vi "CLD 2  Elapsed Time Express Caller Exercise.vi"() -> ()   [LabVIEW 2019]
doc: "CLD 2 Exercise"
panel:
  out "Time Has Elapsed":bool
  out "Elapsed Time (s)":dbl format="%#.2g"
  out "error out":errorcluster
  in  "Time Target (s)":dbl=4.0
  in  "Auto Reset (F)":bool=TRUE
  in  "error in (no error)":errorcluster
  in  "Timer Mode":enum16{"Reset", "Read Status", "Set Auto Reset"}(ring)
  in  "stop":bool
  # "Caller for the FGV"
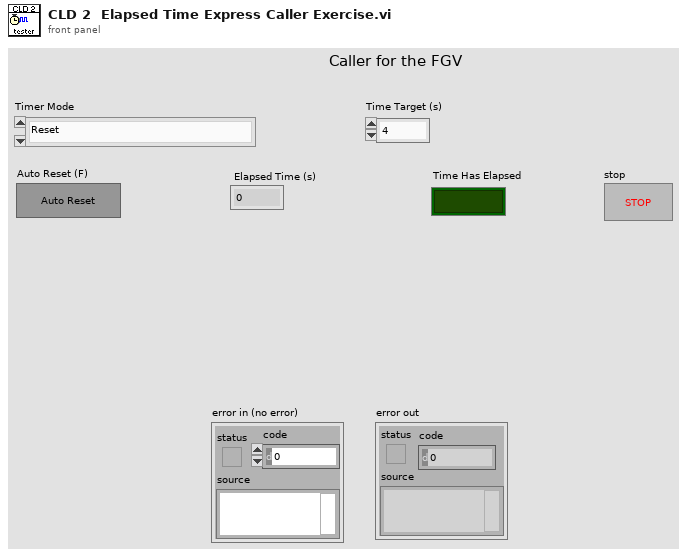
[diagram p1: front panel]
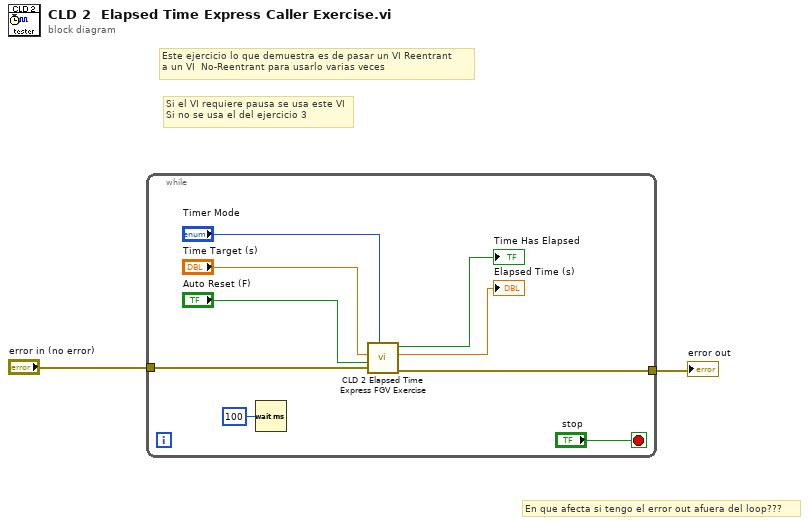
[diagram p0: block diagram]
diagram:
  # "Si el VI requiere pausa se usa este VI\nSi no se usa el del ejercicio 3"
  # "Este ejercicio lo que demuestra es de pasar un VI Reentrant \na un VI  No-Reentrant para usarlo varias veces"
  # "En que afecta si tengo el error out afuera del loop???"
  n1 = while {
    tunnel: "error in (no error)" -> [w10]
    tunnel: [w9] -> w1
    stop <- "stop" stop-if-true
    n2 = Wait (ms)(milliseconds to wait=u32 100) -> ()  [unwired: 1 out]
    n3 = call "CLD 2 Elapsed Time Express FGV Exercise.vi"("Express Timer FGV Enum"="Timer Mode", "error in (no error)"=w10, "Auto Reset (F)"="Auto Reset (F)", "Time Target (s)"="Time Target (s)") -> ("error out"=w9:errorcluster, "Elapsed Time (s)"=→"Elapsed Time (s)":dbl, "Time Has Elapsed"=→"Time Has Elapsed":bool)  [unwired: 5 in]
  }
  "error out" <- w1
